vi "3D Cartesian Coordinate Shift (Scalar).vi"(8 "shift":cluster{"dx":dbl, "dy":dbl, "dz":dbl}, 9 "z":dbl, 10 "y":dbl, 11 "x":dbl) -> (0 "error":i32, 1 "z out":dbl, 2 "y out":dbl, 3 "x out":dbl)   [LabVIEW 2020, in "NI_AALPro.lvlib"]
doc: "Shifts three-dimensional Cartesian coordinates along the x-, y-, and z-axes. \n\nWire data to the <B>X</B> input to determine the polymorphic instance to use or manually select the instance."
uses:
  <vilib>/Analysis/NI_AALPro.lvlib
  <resource>/lvanlys.dll
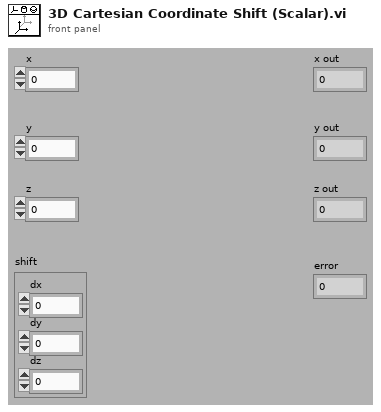
[diagram p1: front panel]
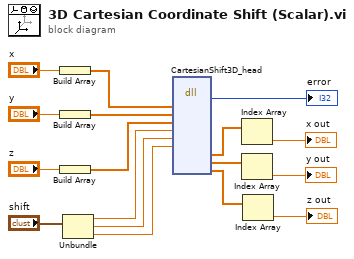
[diagram p0: block diagram]
diagram:
  n1 = Build Array("x") -> (w9:dbl[])
  n2 = Build Array("y") -> (w8:dbl[])
  n3 = Build Array("z") -> (w7:dbl[])
  n4 = Unbundle("shift") -> ("dx"=w16:dbl, "dy"=w15:dbl, "dz"=w14:dbl)
  n5 = dll-call lib="e:/builds/penguin/labview/branches/2020/dev/dist/resource/lvanlys.*" fn="CartesianShift3D_head"("X"=w9, "Y"=w8, "Z"=w7, "dx"=w16, "dy"=w15, "dz"=w14) -> (→"error":i32, "Xout"=w6:dbl[], "Yout"=w4:dbl[], "Zout"=w2:dbl[])  [unwired: 12 in, 2 out]
  n6 = Index Array(array=w6) -> (element=→"x out":dbl)  [unwired: 1 in]
  n7 = Index Array(array=w4) -> (element=→"y out":dbl)  [unwired: 1 in]
  n8 = Index Array(array=w2) -> (element=→"z out":dbl)  [unwired: 1 in]
